vi "Open LabVIEW From CmdLine.vi"(8 "error in (no error)":errorcluster caption="entrée d'erreur (pas d'erreur)", 11 "LabVIEW Version":string) -> (0 "error out":errorcluster caption="sortie d'erreur")   [LabVIEW 2017]
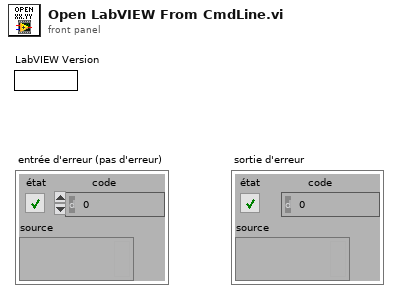
[diagram p1: front panel]
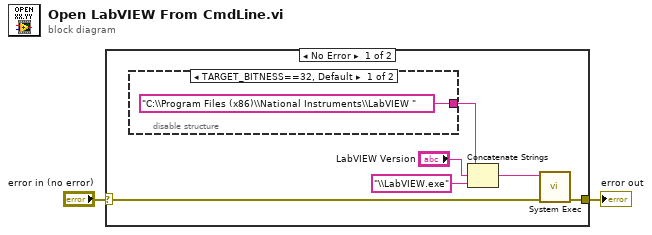
[diagram p0: block diagram]
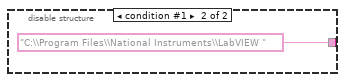
[diagram p2: hidden frame]
diagram:
  n1 = case shown="No Error" "error in (no error)" {
    selector: "error in (no error)" -> [w4 w11]
    tunnel: [w5 w11] -> w2
    frame No Error {
      n2 = disable-structure shown="TARGET_BITNESS==32, Default" {
        disable-tunnel: ["C:\\Program Files (x86)\\National Instruments\\LabVIEW " "C:\\Program Files\\National Instruments\\LabVIEW "] -> w3
        frame condition #0 (active) {
        }
        frame condition #1 {
        }
      }
      n3 = Concatenate Strings(w3, "LabVIEW Version", "\\LabVIEW.exe" ("chaîne")) -> (w6:string)
      n4 = call <vilib>:"System Exec.vi"("error in (no error)"=w4, "command line"=w6) -> ("error out"=w5:errorcluster)  [unwired: 6 in, 3 out]
    }
    frame Error {
    }
  }
  "error out" <- w2
